vi "Interpolation for Y channel.vi"(2 "?":u16(ring)=3 items=["2", "4", "8", "16", "32", "64", "128", "256", "512", "8192", "1024", "2048", "4096", "8192", "16384", "32768", "65536", "131072", "262144", "524288 (one Channel)"], 3 "Sample Duration (sec)":u32(knob)=28 scale=1.0..33.0) -> (0 "array w/ subset deleted":dbl[][](array[numeric]))   [LabVIEW 2010]
uses:
  <vilib>/Analysis/NI_AALPro.lvlib
panel:
  out "size(s)":i32=51
  out "Interpolated Data":dbl[](array[numeric])=[0.20003082713771775, 0.11034679899961915, 0.020662770861520543, -0.06902125727657803, -0.15870528541467666, -0.24838931355277524, -0.33807334169087383, -0.42775736982897244, -0.5174413979670711, -0.6071254261051697, -0.6968094542432682, -0.7864934823813668, -0.7523825350459229, -0.7182715877104788, -0.6841606403750349, -0.6500496930395909, -0.6159387457041469, -0.5818277983687029, -0.5477168510332588, -0.5136059036978149, -0.47949495636237094, -0.4453840090269269, -0.4112730616914829, -0.3162307452739812, -0.2211884288564795, -0.1261461124389773, -0.03110379602147557, 0.06393852039602616, 0.15898083681352787, 0.2540231532310296, 0.3490654696485313, 0.4441077860660335, 0.5391501024835352, 0.634192418901037, 0.9356015136690832, 1.2370106084371293, 1.538419703205177, 1.8398287979732233, 2.1412378927412696, 2.4426469875093155, 2.744056082277362, 3.045465177045408, 3.346874271813456, 3.6482833665815018, 3.949692461349548, 3.9647132873013846, 3.979734113253221, 3.9947549392050576, 4.009775765156895, 4.024796591108731, 4.039817417060568, 4.054838243012404, 4.069859068964241, 4.084879894916077, 4.099900720867914, 4.11492154681975, 3.7674549828900243, 3.419988418960298, 3.072521855030572, 2.7250552911008463, 2.3775887271711205, 2.030122163241391, 1.682655599311665, 1.335189035381939, 0.9877224714522129, 0.640255907522487, 0.292789343592761, 0.3107378892509554, 0.3286864349091499, 0.3466349805673443, 0.36458352622553875, 0.38253207188373317, 0.4004806175419278, 0.41842916320012224, 0.43637770885831667, 0.4543262545165111, 0.4722748001747056, 0.4902233458329, 0.6694459722196231, 0.8486685986063461, 1.0278912249930692, 1.2071138513797923, 1.3863364777665153, 1.5655591041532402, 1.7447817305399633, 1.9240043569266863, 2.103226983313409, 2.2824496097001323, 2.4616722360868555, 2.3592214905277267, 2.2567707449686, 2.1543199994094713, 2.0518692538503447, 1.9494185082912159, 1.846967762732089, 1.7445170171729605, 1.6420662716138337, 1.5396155260547049, 1.4371647804955783, 1.3347140349364495, 0.8573655010725375, 0.38001696720863487, -0.09733156665527706, -0.5746801005191797, -1.0520286343830916, -1.5293771682469943, -2.006725702110906, -2.4840742359748087, -2.961422769838721, -3.4387713037026235, -3.9161198375665354, -3.90101145702002, -3.8859030764735047, -3.8707946959269894, -3.855686315380474, -3.840577934833959, -3.825469554287444, -3.8103611737409286, -3.7952527931944133, -3.780144412647898, -3.7650360321013827, -3.7499276515548674, -3.4575984773832897, -3.1652693032117174, -2.8729401290401397, -2.580610954868568, -2.28828178069699, -1.995952606525418, -1.7036234323538402, -1.4112942581822683, -1.1189650840106904, -0.8266359098391184, -0.5343067356675406, -0.5745957077601763, -0.6148846798528111, -0.6551736519454469, -0.6954626240380818, -0.7357515961307174, -0.7760405682233523, -0.8163295403159879, -0.8566185124086229, -0.8969074845012586, -0.9371964565938934, -0.9774854286865291, -1.2676479506691007, -1.5578104726516666, -1.8479729946342383, -2.138135516616804, -2.428298038599376, -2.7184605605819416, -3.0086230825645135, -3.298785604547079, -3.588948126529651, -3.879110648512217, -4.1692731704947885, -4.015847101966035, -3.8624210334372844, -3.708994964908531, -3.5555688963797802, -3.402142827851027, -3.2487167593222765, -3.095290690793523, -2.9418646222647724, -2.788438553736019, -2.6350124852072683, -2.481586416678515, -2.134093693178331, -1.786600969678154, -1.43910824617797, -1.0916155226777928, -0.7441227991776089, -0.39663007567743186, -0.049137352177247975, 0.2983553713229291, 0.645848094823113, 0.9933408183232901, 1.340833541823474, 1.322679987332474, 1.3045264328414732, 1.286372878350473, 1.268219323859473, 1.250065769368473, 1.231912214877472, 1.2137586603864718, 1.1956051058954718, 1.1774515514044717, 1.159297996913471, 1.1411444424224708, 1.0324575996667698, 0.9237707569110645, 0.8150839141553634, 0.7063970713996625, 0.5977102286439614, 0.48902338588825606, 0.38033654313255505, 0.271649700376854, 0.16296285762115295, 0.05427601486544766, -0.05441082789025338, 0.0195793375573303, 0.09356950300491687, 0.16755966845250056, 0.24154983390008422, 0.3155399993476679, 0.3895301647952545, 0.4635203302428382, 0.5375104956904219, 0.6115006611380055, 0.6854908265855921, 0.7594809920331758, 0.8855897502152605, 1.0116985083973502, 1.1378072665794348, 1.2639160247615195, 1.3900247829436043, 1.516133541125694, 1.6422422993077788, 1.7683510574898635, 1.894459815671948, 2.020568573854038, 2.1466773320361225, 2.1319787579627993, 2.1172801838894753, 2.102581609816152, 2.087883035742829, 2.0731844616695057, 2.0584858875961816, 2.0437873135228584, 2.029088739449535, 2.0143901653762115, 1.9996915913028876, 1.9849930172295644, 1.8397060334735431, 1.6944190497175162, 1.549132065961495, 1.4038450822054738, 1.2585580984494524, 1.1132711146934255, 0.9679841309374043, 0.822697147181383, 0.6774101634253618, 0.5321231796693349, 0.3868361959133136, 0.18585975575295627, -0.015116684407408909, -0.21609312456776622, -0.41706956472812357, -0.6180460048884808, -0.819022445048846, -1.0199988852092035, -1.2209753253695608, -1.421951765529918, -1.6229282056902832, -1.8239046458506405, -1.7850504137980816, -1.7461961817455214, -1.7073419496929625, -1.6684877176404036, -1.629633485587845, -1.5907792535352845, -1.5519250214827258, -1.513070789430167, -1.474216557377608, -1.4353623253250478, -1.396508093272489, -1.2449851876300846, -1.0934622819876745, -0.9419393763452703, -0.790416470702866, -0.6388935650604618, -0.4873706594180516, -0.3358477537756473, -0.18432484813324307, -0.03280194249083882, 0.11872096315157135, 0.2702438687939756, 0.08484428873356772, -0.10055529132684739, -0.2859548713872553, -0.47135445144766314, -0.656754031508071, -0.8421536115684861, -1.027553191628894, -1.2129527716893018, -1.3983523517497098, -1.583751931810125, -1.7691515118705328, -1.7707033386692226, -1.7722551654679126, -1.7738069922666024, -1.7753588190652922, -1.7769106458639823, -1.778462472662672, -1.7800142994613621, -1.781566126260052, -1.7831179530587418, -1.7846697798574318, -1.7862216066561216, -1.578540069158614, -1.3708585316610984, -1.1631769941635908, -0.9554954566660833, -0.7478139191685756, -0.54013238167106, -0.3324508441735524, -0.12476930667604487, 0.08291223082146269, 0.2905937683189784, 0.49827530581648594, 0.3434144459484374, 0.18855358608038283, 0.033692726212334316, -0.12116813365571422, -0.27602899352376276, -0.4308898533918173, -0.5857507132598658, -0.7406115731279144, -0.8954724329959629, -1.0503332928640174, -1.205194152732066, -1.3208784560413236, -1.4365627593505856, -1.552247062659843, -1.6679313659691006, -1.7836156692783582, -1.89929997258762, -2.014984275896878, -2.130668579206135, -2.2463528825153927, -2.3620371858246547, -2.4777214891339123, -2.3334601348523005, -2.1891987805706834, -2.0449374262890716, -1.9006760720074602, -1.7564147177258487, -1.6121533634442313, -1.4678920091626197, -1.3236306548810082, -1.1793693005993964, -1.0351079463177792, -0.8908465920361676, -0.8122303534413046, -0.7336141148464385, -0.6549978762515755, -0.5763816376567125, -0.4977653990618494, -0.4191491604669833, -0.3405329218721203, -0.26191668327725726, -0.18330044468239426, -0.10468420608752817, -0.026067967492665153, -0.21126251996614911, -0.3964570724396186, -0.5816516249131026, -0.7668461773865866, -0.9520407298600561, -1.13723528233354, -1.3224298348070096, -1.5076243872804935, -1.6928189397539775, -1.878013492227447, -2.063208044700931, -1.974109751877879, -1.885011459054834, -1.795913166231782, -1.70681487340873, -1.617716580585685, -1.528618287762633, -1.439519994939588, -1.3504217021165361, -1.2613234092934842, -1.1722251164704391, -1.0831268236473872, -1.0289299596569768, -0.9747330956665705, -0.9205362316761602, -0.8663393676857497, -0.8121425036953435, -0.757945639704933, -0.7037487757145268, -0.6495519117241163, -0.595355047733706, -0.5411581837432997, -0.48696131975288925, -0.6212968730186699, -0.7556324262844399, -0.8899679795502206, -1.024303532816001, -1.1586390860817712, -1.2929746393475519, -1.427310192613322, -1.5616457458791027, -1.695981299144883, -1.8303168524106532, -1.9646524056764338, -1.9634812156702013, -1.962310025663969, -1.9611388356577366, -1.959967645651504, -1.9587964556452717, -1.9576252656390392, -1.9564540756328068, -1.9552828856265743, -1.954111695620342, -1.9529405056141096, -1.951769315607877, -1.714866533416412, -1.4779637512249655, -1.2410609690335004, -1.0041581868420353, -0.7672554046505888, -0.5303526224591238, -0.2934498402676773, -0.056547058076212256, 0.18035572411525277, 0.4172585063066993, 0.6541612884981644, 0.40490245173379696, 0.15564361496944903, -0.09361522179491837, -0.34287405855928577, -0.5921328953236337, -0.8413917320880011, -1.090650568852349, -1.3399094056167165, -1.5891682423810838, -1.8384270791454318, -2.087685915909799, -2.3575285946009887, -2.6273712732921575, -2.897213951983347, -3.1670566306745367, -3.436899309365705, -3.706741988056895, -3.9765846667480633, -4.246427345439253, -4.516270024130443, -4.786112702821611, -5.055955381512801, -4.645862646639058, -4.235769911765348, -3.825677176891605, -3.4155844420178627, -3.0054917071441523, -2.59539897227041, -2.185306237396699, -1.7752135025229565, -1.365120767649214, -0.9550280327755035, -0.544935297901761, -0.2659270028936205, 0.013081292114498173, 0.29208958712263866, 0.5710978821307792, 0.8501061771388978, 1.1291144721470383, 1.408122767155157, 1.6871310621632976, 1.9661393571714378, 2.245147652179557, 2.524155947187697, 2.2285752959959066, 1.932994644804139, 1.6374139936123484, 1.3418333424205577, 1.0462526912287902, 0.7506720400369996, 0.45509138884523215, 0.1595107376534415, -0.13606991353834907, -0.4316505647301166, -0.7272312159219072, -0.7891579193810847, -0.8510846228402574, -0.9130113262994349, -0.9749380297586124, -1.0368647332177852, -1.0987914366769627, -1.1607181401361353, -1.2226448435953128, -1.2845715470544905, -1.3464982505136631, -1.4084249539728406, -1.007407323111525, -0.6063896922502406, -0.20537206138892497, 0.19564556947239067, 0.596663200333675, 0.9976808311949906, 1.398698462056275, 1.7997160929175906, 2.200733723778906, 2.6017513546401907, 3.0027689855015063, 3.208229483623957, 3.4136899817463915, 3.619150479868842, 3.8246109779912927, 4.0300714761137275, 4.235531974236178, 4.440992472358612, 4.646452970481063, 4.851913468603514, 5.057373966725948, 5.262834464848399, 4.9622136773422385, 4.661592889836101, 4.360972102329941, 4.060351314823781, 3.759730527317645, 3.4591097398114847, 3.158488952305348, 2.857868164799188, 2.5572473772930278, 2.256626589786891, 1.9560058022807307, 1.6536620315581363, 1.3513182608355654, 1.048974490112971, 0.7466307193903765, 0.4442869486678056, 0.14194317794521114, -0.16040059277735969, -0.4627443634999542, -0.7650881342225486, -1.0674319049451195, -1.369775675667714, -1.3555164332893206, -1.3412571909109283, -1.326997948532535, -1.3127387061541416, -1.2984794637757493, -1.2842202213973561, -1.2699609790189639, -1.2557017366405705, -1.2414424942621771, -1.2271832518837849, -1.2129240095053915, -1.129593763626276, -1.046263517747167, -0.9629332718680517, -0.8796030259889362, -0.7962727801098274, -0.7129425342307119, -0.629612288351603, -0.5462820424724876, -0.4629517965933721, -0.3796215507142632, -0.29629130483514776, -0.2693557316683154, -0.2424201585014851, -0.21548458533465273, -0.18854901216782036, -0.16161343900099007, -0.1346778658341577, -0.10774229266732742, -0.08080671950049503, -0.053871146333662655, -0.02693557316683238, 0.0] format="%0.2f"
  out "Raw Data and Interpolated Data":cluster{dbl[], "Best Exponential Fit":dbl[]}[](graph)=[{[0.0, 1.0, 2.0, 3.0, 4.0, 5.0, 6.0, 7.0, 8.0, 9.0, 10.0, 11.0, 12.0, 13.0, 14.0, 15.0, 16.0, 17.0, 18.0, 19.0, 20.0, 21.0, 22.0, 23.0, 24.0, 25.0, 26.0, 27.0, 28.0, 29.0, 30.0, 31.0, 32.0, 33.0, 34.0, 35.0, 36.0, 37.0, 38.0, 39.0, 40.0, 41.0, 42.0, 43.0, 44.0, 45.0, 46.0, 47.0, 48.0, 49.0, 50.0, 51.0], "Best Exponential Fit"=[0.20003082713771775, -0.7864934823813668, -0.4112730616914829, 0.634192418901037, 3.949692461349548, 4.11492154681975, 0.292789343592761, 0.4902233458329, 2.4616722360868555, 1.3347140349364495, -3.9161198375665354, -3.7499276515548674, -0.5343067356675406, -0.9774854286865291, -4.1692731704947885, -2.481586416678515, 1.340833541823474, 1.1411444424224708, -0.05441082789025338, 0.7594809920331758, 2.1466773320361225, 1.9849930172295644, 0.3868361959133136, -1.8239046458506405, -1.396508093272489, 0.2702438687939756, -1.7691515118705328, -1.7862216066561216, 0.49827530581648594, -1.205194152732066, -2.4777214891339123, -0.8908465920361676, -0.026067967492665153, -2.063208044700931, -1.0831268236473872, -0.48696131975288925, -1.9646524056764338, -1.951769315607877, 0.6541612884981644, -2.087685915909799, -5.055955381512801, -0.544935297901761, 2.524155947187697, -0.7272312159219072, -1.4084249539728406, 3.0027689855015063, 5.262834464848399, 1.9560058022807307, -1.369775675667714, -1.2129240095053915, -0.29629130483514776, 0.0]}, {array[562 elements], "Best Exponential Fit"=array[562 elements]}]
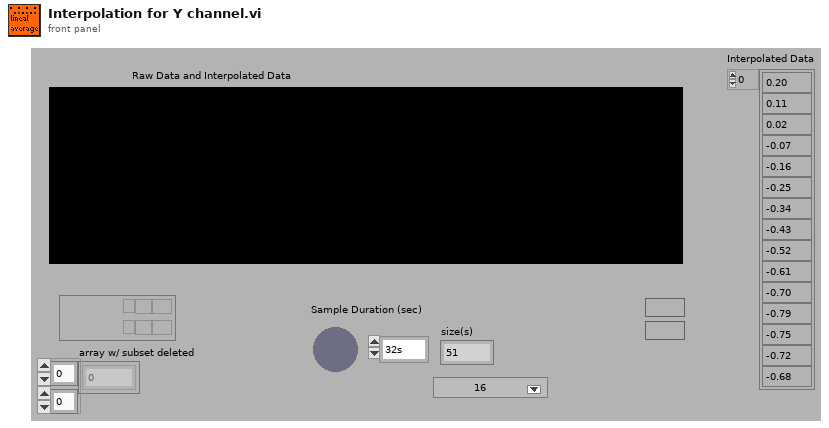
[diagram p1: front panel]
types:
  T1 = enum16{"Linear", "Polynomial", "Spline", "Rational"}
  T2 = cluster{"Type of Interpolation":enum16{"Linear", "Polynomial", "Spline", "Rational"}, "Points Between":i32}
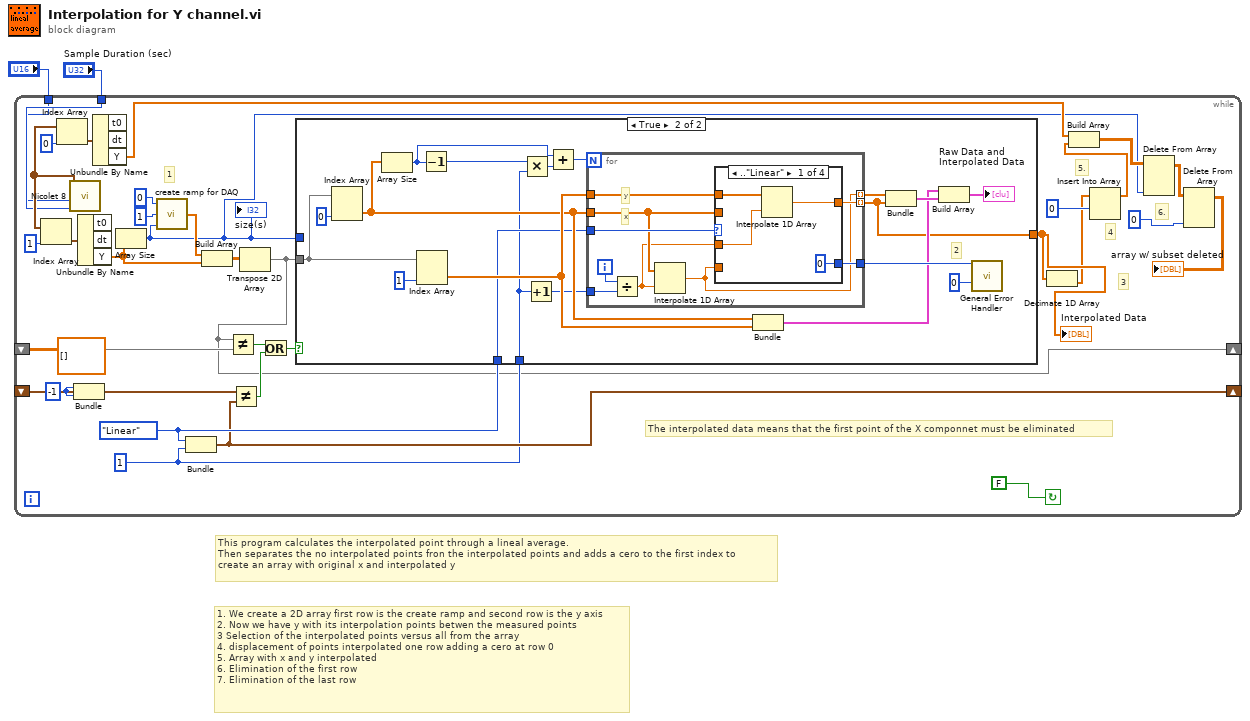
[diagram p0: block diagram]
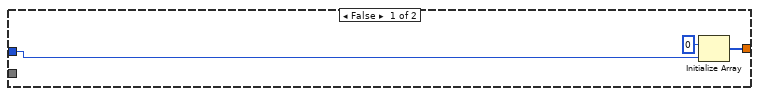
[diagram p2: hidden frame]
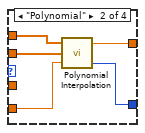
[diagram p3: hidden frame]
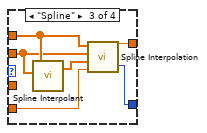
[diagram p4: hidden frame]
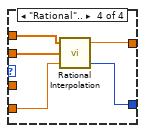
[diagram p5: hidden frame]
diagram:
  w3 = -1
  # "1. We create a 2D array first row is the create ramp and second row is the y axis\n2. Now we have y with its interpolation points betwen the measured points\n3 Selection of the interpolated points versus all from the array\n4. displacement of points interpolated one row adding a cero at row 0\n5. Array with x and y interpolated\n6. Elimination of the first row\n7. Elimination of the last row"
  # "This program calculates the interpolated point through a lineal average. \nThen separates the no interpolated points fron the interpolated points and adds a cero to the first index to \ncreate an array with original x and interpolated y"
  n1 = Bundle(w3, w3) -> (w4:cluster{i32, i32})  [unwired: 1 out]
  n2 = while {
    shift-left: w4 -> [w32]
    shift-right: [w31] -> _
    shift-left: dbl[][] [] -> [w37]
    shift-right: [w22] -> _
    tunnel: "Sample Duration (sec)" -> [w7]
    tunnel: "?" -> [w6]
    stop <- FALSE ("stop") continue-if-true
    w33 = T1."Linear" ("Type of Interpolation")
    w29 = 1 ("Points Between")
    w16 = 0
    # "6."
    # "5."
    # "4"
    # "3"
    # "1"
    # "The interpolated data means that the first point of the X componnet must be eliminated"
    n3 = call "Nicolet 8.vi"(3:w6, "Sample Duration (sec)"=w7) -> ("Waveform Graph"=w19:waveform(dbl)[])  [unwired: 6 out]
    n4 = Index Array(array=w19, index=1) -> (element=w27:waveform(dbl))
    n5 = Index Array(array=w19, index=0) -> (element=w18:waveform(dbl))
    n6 = Unbundle By Name(w27) -> ("Y"=w14:dbl[])  [unwired: 2 out]
    n7 = Unbundle By Name(w18) -> ("Y"=w17:dbl[])  [unwired: 2 out]
    n8 = Array Size(array=w14) -> (size(s)=w10:i32)
    "size(s)" <- w10
    n9 = call "create ramp for DAQ.vi"("final value"=w10, "increment"=1, "starting value"=0) -> ("ramp data"=w24:dbl[])
    n10 = Bundle("Type of Interpolation"=w33, "Points Between"=w29) -> (w31:T2)  [unwired: 1 out]
    n11 = Build Array(w24, w14) -> (w23:dbl[][])
    n12 = Not Equal?(x=w32, y=w31) -> (x != y?=w35:bool)
    n13 = Transpose 2D Array(2D array=w23) -> (transposed array=w22:dbl[][])
    n14 = Not Equal?(x=w22, y=w37) -> (x != y?=w36:bool)
    n15 = Or(x=w36, y=w35) -> (x .or. y?=w34:bool)
    n16 = case shown="True" w34 {
      tunnel: w22 -> [_ w52]
      tunnel: w33 -> [_ w44]
      tunnel: w29 -> [_ w43]
      tunnel: [w40 w41] -> w21
      tunnel: w10 -> [w38 _]
      frame False {
        n17 = Initialize Array(0, w38) -> (w40:i32[])
      }
      frame True {
        # "2"
        n18 = Index Array(array=w52, index (col)=0) -> (element=w50:dbl[])  [unwired: 1 in]
        n19 = Array Size(array=w50) -> (size(s)=w46:i32)
        n20 = Index Array(array=w52, index (col)=1) -> (element=w51:dbl[])  [unwired: 1 in]
        n21 = Decrement(x=w46) -> (x-1=w49:i32)
        n22 = Multiply(x=w49, y=w43) -> (x*y=w47:i32)
        n23 = Increment(x=w43) -> (x+1=w48:i32)
        n24 = Add(x=w46, y=w47) -> (x+y=w45:i32)
        n25 = for {
          N: w45 -> [_]
          tunnel: w51 -> [w68]
          tunnel: w50 -> [w62]
          tunnel: [w67] -> w59
          tunnel: w44 -> [w63]
          tunnel: w48 -> [w65]
          tunnel: [w64] -> w41 mode=indexing
          tunnel: [w61] -> w42 mode=indexing
          i -> [w66]
          # "x"
          # "y"
          n26 = Divide(x=w66, y=w65) -> (x/y=w60:dbl)
          n27 = Interpolate 1D Array(1:w60, 2:w62) -> (0:w61:dbl)
          n28 = case shown="..\"Linear\"" w63 {
            tunnel: w61 -> [_ w77 w80 w84]
            tunnel: [w71 w76 w78 w86] -> w64
            tunnel: [0 w75 w79 w85] -> w67
            tunnel: w62 -> [_ w74 w81 w87]
            tunnel: w68 -> [w72 w73 w83 w88]
            tunnel: w60 -> [w69 _ _ _]
            frame .."Linear" {
              n29 = Interpolate 1D Array(1:w69, 2:w72) -> (0:w71:dbl)
            }
            frame "Polynomial" {
              n30 = call <vilib>:"Polynomial Interpolation.vi"("x value"=w77, "X"=w74, "Y"=w73) -> ("error"=w75:i32, "interpolation value"=w76:dbl)  [unwired: 1 out]
            }
            frame "Spline" {
              n31 = call <vilib>:"Spline Interpolant.vi"("X"=w81, "Y"=w83) -> ("Interpolant"=w82:dbl[])  [unwired: 2 in, 1 out]
              n32 = call <vilib>:"Spline Interpolation.vi"("x value"=w80, "Interpolant"=w82, "X"=w81, "Y"=w83) -> ("error"=w79:i32, "interpolation value"=w78:dbl)
            }
            frame "Rational".. {
              n33 = call <vilib>:"Rational Interpolation.vi"("x value"=w84, "X"=w87, "Y"=w88) -> ("error"=w85:i32, "interpolation value"=w86:dbl)  [unwired: 1 out]
            }
          }
        }
        n34 = Bundle(w50, w51) -> (w54:cluster{dbl[], dbl[]})  [unwired: 1 out]
        n35 = Bundle(w42, w41) -> (w58:cluster{dbl[], dbl[]})  [unwired: 1 out]
        n36 = Build Array(w54, w58) -> (→"Raw Data and Interpolated Data":cluster{dbl[], dbl[]}[])
        n37 = call <vilib>:"General Error Handler.vi"("[error code] (0)"=w59, "type of dialog (OK msg:1)"=0) -> ()  [unwired: 1 in, 13 out]
      }
    }
    "Interpolated Data" <- w21
    n38 = Decimate 1D Array(w21) -> (w15:dbl[])  [unwired: 1 out]
    n39 = Insert Into Array(array=w15, index=w16, new element=w16) -> (w13:dbl[])
    n40 = Build Array(w17, w13) -> (w12:dbl[][])
    n41 = Delete From Array(array=w12, index (col)=w10) -> (array with subset deleted=w9:dbl[][])  [unwired: 2 in, 1 out]
    n42 = Delete From Array(array=w9, index (col)=0) -> (array with subset deleted=→"array w/ subset deleted":dbl[][])  [unwired: 2 in, 1 out]
  }
